vi "Bodies_GetPtVInXYZ0.vi"(8 "error in (no error)":errorcluster, 9 "Joint V":dbl[](array[numeric]), 10 "Point":T1, 11 "Bodies.lvclass":refnum<class "Bodies.lvclass">) -> (0 "error out":errorcluster, 1 "Pt In GCS":dbl[](array[numeric]) format="%#.6f", 2 "Pt V InGCS":dbl[](array[numeric]), 3 "Bodies.lvclass 2":refnum<class "Bodies.lvclass">)   [LabVIEW 2015, in "Bodies.lvclass"]
uses:
  Bodies.lvclass
  PointOnBody.ctl
  Bodies.lvclass/Bodies.ctl
  <vilib>/Analysis/Matrix/Numeric/Conversions/Array To Matrix - RA2.vi
  <vilib>/Analysis/BLAS.llb/dgemv - General Matrix-Vector Product (DBL).vi
  <vilib>/Analysis/NI_AALBLAS.lvlib
  <vilib>/Analysis/NI_AALBase.lvlib
  <vilib>/Analysis/Matrix/NI_Matrix.lvlib
  <vilib>/Analysis/baseanly.llb/A x Vector.vi
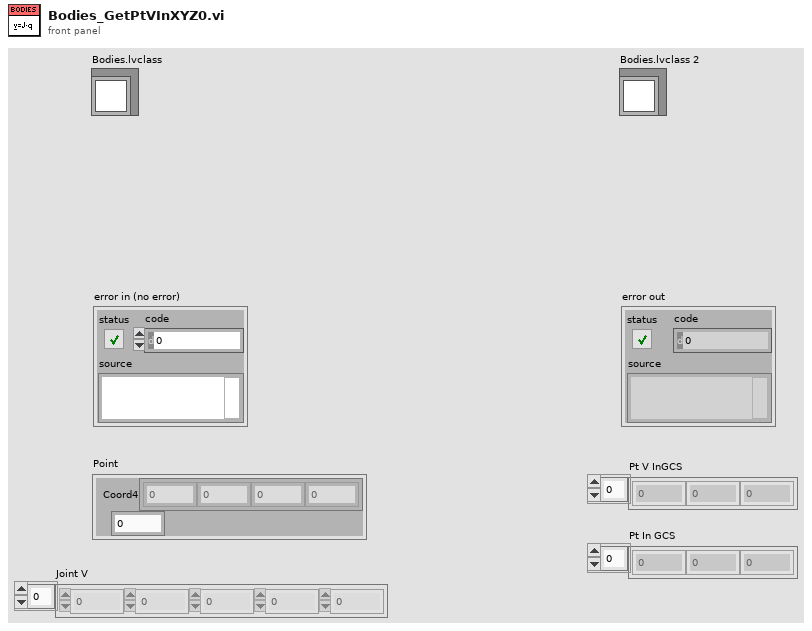
[diagram p1: front panel]
types:
  T1 = typedef "Bodies.lvclass/PointOnBody.ctl" = cluster{"Coord4":dbl[], "ID":i32}
  T2 = typedef "NI_Matrix.lvlib/RealMatrix.ctl" = dbl[][]
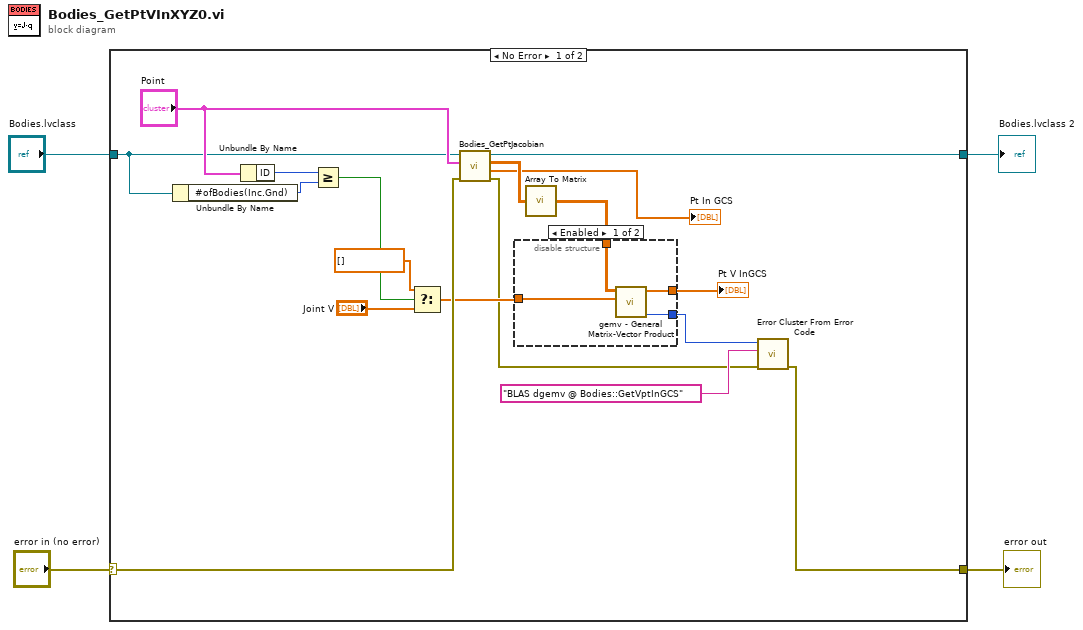
[diagram p0: block diagram]
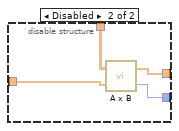
[diagram p2: hidden frame]
diagram:
  n1 = case shown="No Error" "error in (no error)" {
    selector: "error in (no error)" -> [w19 w32]
    tunnel: "Bodies.lvclass" -> [w9 w31]
    tunnel: [w22 w32] -> w3
    tunnel: [w18 w31] -> w1
    frame No Error {
      n2 = Unbundle By Name(w9) -> ("#ofBodies(Inc.Gnd)"=w11:i32)
      n3 = Unbundle By Name("Point") -> ("ID"=w8:i32)
      n4 = Greater Or Equal?(x=w8, y=w11) -> (x >= y?=w12:bool)
      n5 = Select(t=dbl[] [], s=w12, f="Joint V") -> (s? t:f=w6:dbl[])
      n6 = call "Bodies_GetPtJacobian.vi"("error in (no error)"=w19, "Point"="Point", "Bodies.lvclass"=w9) -> ("error out"=w5:errorcluster, "PointInGCS"=→"Pt In GCS":dbl[], "Jacobian"=w17:dbl[][], "Bodies.lvclass 2"=w18:refnum<class "Bodies.lvclass">)  [unwired: 5 in]
      n7 = call-poly <vilib>:"Array To Matrix.vi"("Real 2D Array"=w17) -> ("Real Matrix"=w16:T2)
      n8 = disable-structure shown="Enabled" {
        disable-tunnel: [w26 w27] -> w20
        disable-tunnel: [w24 w28] -> w15
        disable-tunnel: w16 -> [w25 w30]
        disable-tunnel: w6 -> [w23 w29]
        frame Enabled {
          n9 = call-poly <vilib>:"gemv - General Matrix-Vector Product.vi"("x"=w23, "A"=w25) -> ("error"=w26:i32, "dgemv"=w24:dbl[])  [unwired: 8 in]
        }
        frame Disabled {
          n10 = call-poly <vilib>:"A x B.vi"("Vector"=w29, "A"=w30) -> ("error"=w27:i32, "A x Vector"=w28:dbl[])
        }
      }
      "Pt V InGCS" <- w15
      n11 = call <vilib>:"Error Cluster From Error Code.vi"("error in (no error)"=w5, "error message (\"\")"="BLAS dgemv @ Bodies::GetVptInGCS" ("error source (\" \")"), "error code (0)"=w20) -> ("error out"=w22:errorcluster)  [unwired: 6 in]
    }
    frame Error {
    }
  }
  "error out" <- w3
  "Bodies.lvclass 2" <- w1
